vi "Path_GV.vi"() -> ()   [LabVIEW 2016]
panel:
  out "Logger Save Folder":path=path "C:/CAlexExpData"
  out "MTP Folder":path=path "c:/MotorParam"
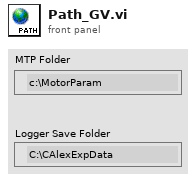
[diagram p1: front panel]
diagram:
